vi "shut-down.vi"(8 "error in (no error)":errorcluster, 11 "GenericToplevelComponent in":refnum<class "GenericToplevelComponent.lvclass">) -> (0 "error out":errorcluster, 3 "GenericToplevelComponent out":refnum<class "GenericToplevelComponent.lvclass">)   [LabVIEW 2010, in "GenericToplevelComponent.lvclass"]
uses:
  GenericToplevelComponent.lvclass
  ErrorController/ErrorController/class_data.vi
  ErrorController/ErrorController/ErrorController.lvclass
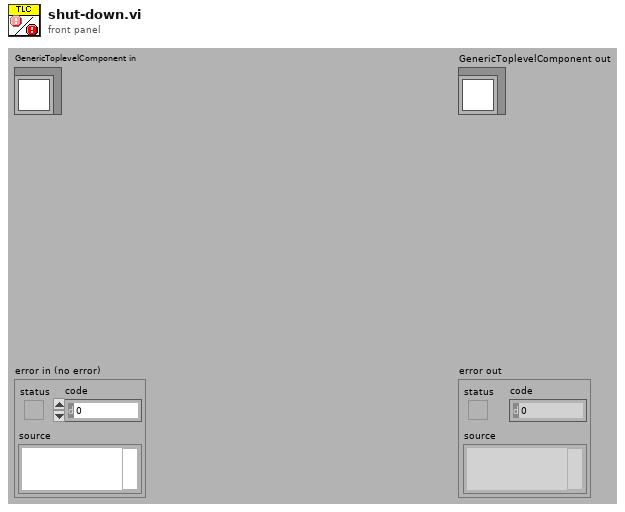
[diagram p1: front panel]
types:
  T1 = typedef "GenericToplevelComponent.lvclass/common_trigger_enum.ctl" = enum16{"NULL", "initialise", "terminate", "fetch command", "fetch data", "attach observer", "register as observer", "detach observer", "acknowledge", "start", "stop", "sweep started", "sweep finished", "experiment started", "experiment stopped"}
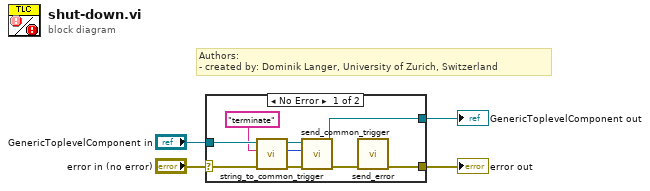
[diagram p0: block diagram]
diagram:
  # "Authors: \n- created by: Dominik Langer, University of Zurich, Switzerland"
  n1 = case shown="No Error" "error in (no error)" {
    selector: "error in (no error)" -> [w12 w15]
    tunnel: [w13 w15] -> w3
    tunnel: [w6 w14] -> w1
    tunnel: "GenericToplevelComponent in" -> [w11 w14]
    frame No Error {
      n2 = call-dynamic "string_to_common_trigger.vi"("error in (no error)"=w12, "trigger string"="terminate", "GenericToplevelComponent in"=w11) -> ("error out"=w8:errorcluster, "trigger"=w9:T1, "GenericToplevelComponent out"=w10:refnum<class "GenericToplevelComponent.lvclass">)  [unwired: 6 in]
      n3 = call-dynamic "send_common_trigger.vi"("error in (no error)"=w8, "trigger"=w9, "GenericToplevelComponent in"=w10) -> ("error out"=w5:errorcluster, "GenericToplevelComponent out"=w6:refnum<class "GenericToplevelComponent.lvclass">)  [unwired: 6 in, 1 out]
      n4 = call "send_error.vi"("error in (no error)"=w5) -> ("error out"=w13:errorcluster)  [unwired: 10 in]
    }
    frame Error {
    }
  }
  "error out" <- w3
  "GenericToplevelComponent out" <- w1
